vi "Controller Generate Filter Coefficients.vi"(4 "Destination Folder":path, 5 "iwl coeff b":i16=2, 6 "Filter Name":string, 7 "iwl coeff a":i16=2, 8 "Generate FPGA Code?":bool, 9 "wl":i16=20, 10 "denominator":dbl[](array[numeric]), 11 "numerator":dbl[](array[numeric])) -> (1 "gain":dbl, 2 "coeff a":dbl[](array[numeric]), 3 "coeff b":dbl[](array[numeric]))   [LabVIEW 2011]
uses:
  <vilib>/addons/Digital Filter Design/_Objects.llb/DFD Output Iwl Obj.ctl
  <vilib>/addons/Digital Filter Design/_Objects.llb/DFD Quantization Settings.ctl
  <vilib>/addons/Digital Filter Design/_Objects.llb/DFD Quantization Sources.ctl
  <vilib>/addons/Digital Filter Design/_Objects.llb/DFD Phase Setting.ctl
  <vilib>/addons/Digital Filter Design/_Objects.llb/DFD Coef Norm Type.ctl
  <vilib>/addons/Digital Filter Design/FXPModel.llb/DFD FXP Quantize Coef (Advanced).vi
  <vilib>/addons/Digital Filter Design/NI_DigFilterLicensed.lvlib
  <vilib>/addons/Digital Filter Design/CodeGen.llb/DFD FXP LabVIEW FPGA Code Generator.vi
panel:
  out "max gain error (dB)":dbl
  out "max phase error (deg)":dbl
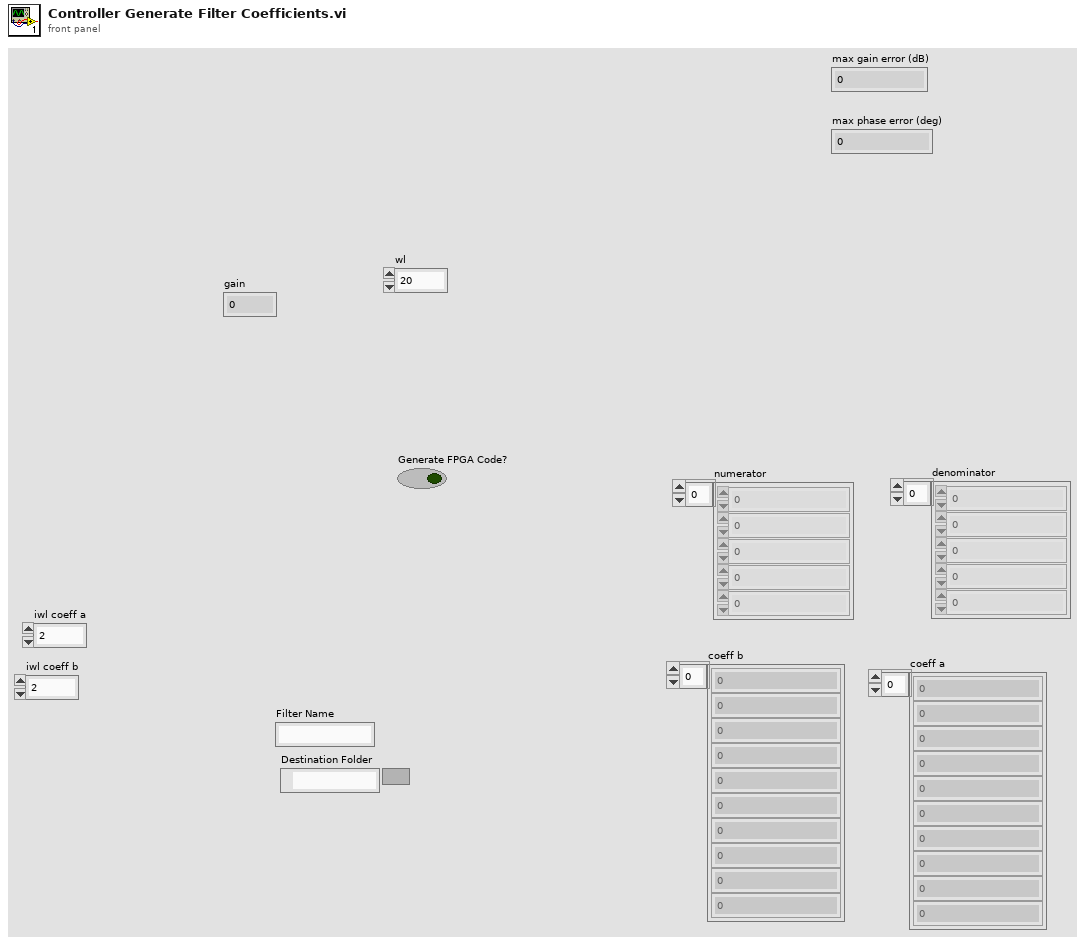
[diagram p1: front panel]
types:
  T1 = typedef "NI_DigFilterLicensed.lvlib/DFD Coef Norm Type.ctl" = enum16{"No Norm", "Time Domain 1-Norm", "Time Domain 2-Norm", "Time Domain Inf-Norm"}
  T2 = typedef "NI_DigFilterLicensed.lvlib/DFD Phase Setting.ctl" = cluster{"unwrap? (F)":bool, "degree? (F)":bool}
  T3 = typedef "NI_DigFilterLicensed.lvlib/DFD Quantization Settings.ctl" = cluster{"source":T4, "wl":i16, "iwl":i16, "overflow mode":enum16{"Saturation", "Wrap"}, "rounding mode":enum16{"Nearest", "Truncation"}, "signed?":bool}
  T4 = typedef "NI_DigFilterLicensed.lvlib/DFD Quantization Sources.ctl" = u16
  T5 = typedef "NI_DigFilterLicensed.lvlib/DFD Output Iwl Obj.ctl" = cluster{"output option":enum16{"Auto", "Same As Input", "User Defined"}, "integer word length":i16}
  T6 = typedef "NI_DigFilterLicensed.lvlib/DFD Filter Obj.ctl" = cluster{"mSRate_Fs":dbl, "mSRate_Version":string, "mSRate_Comments":string, "mSRate_OrgCoef":T7, "mSRate_CurCoef":T7, "mSRate_Quantized?":bool, "mSRate_QCoef":T7, "mSRate_QSettings":T9[], "mSRate_Order":i32, "mSRate_Scaling":cluster{"mSRate_ScaleByPowerOf2?":bool, "mSRate_ScaleType":T1}}
  T7 = typedef "NI_DigFilterLicensed.lvlib/DFD Filter Coef.ctl" = cluster{"type":T8, "gain":dbl, "coef a (k)":dbl[], "coef b (v)":dbl[]}
  T8 = typedef "NI_DigFilterLicensed.lvlib/DFD Filter Structure Type Selector.ctl" = enum16{"Undefined", "FIR Direct Form", "FIR Direct Form Transposed", "FIR Symmetric", "FIR Antisymmetric", "IIR Direct Form I", "IIR Direct Form I Transposed", "IIR Direct Form II", "IIR Direct Form II Transposed", "IIR Cascaded Second Order Sections Form I", "IIR Cascaded Second Order Sections Form I Transposed", "IIR Cascaded Second Order Sections Form II", "IIR Cascaded Second Order Sections Form II Transposed", "Lattice Allpass (basic sections)", "Lattice Allpass (one multiplier sections)", "Lattice Allpass (normalized sections)", "Lattice AR (basic sections)", "Lattice AR (one multiplier sections)", "Lattice AR (normalized sections)", "Lattice MA (minimum phase)", "Lattice MA (maximum phase)", "Lattice ARMA (basic sections)", "Lattice ARMA (one multiplier sections)", "Lattice ARMA (normalized sections)"}
  T9 = typedef "NI_DigFilterLicensed.lvlib/dfd_Internal Quantization Settings.ctl" = cluster{"source":T10, "wl":i16, "iwl":i16, "overflow mode":enum16{"Saturation", "Wrap"}, "rounding mode":enum16{"Nearest", "Truncation"}, "signed?":bool}
  T10 = typedef "NI_DigFilterLicensed.lvlib/dfd_Internal Quantization Srcs.ctl" = u16
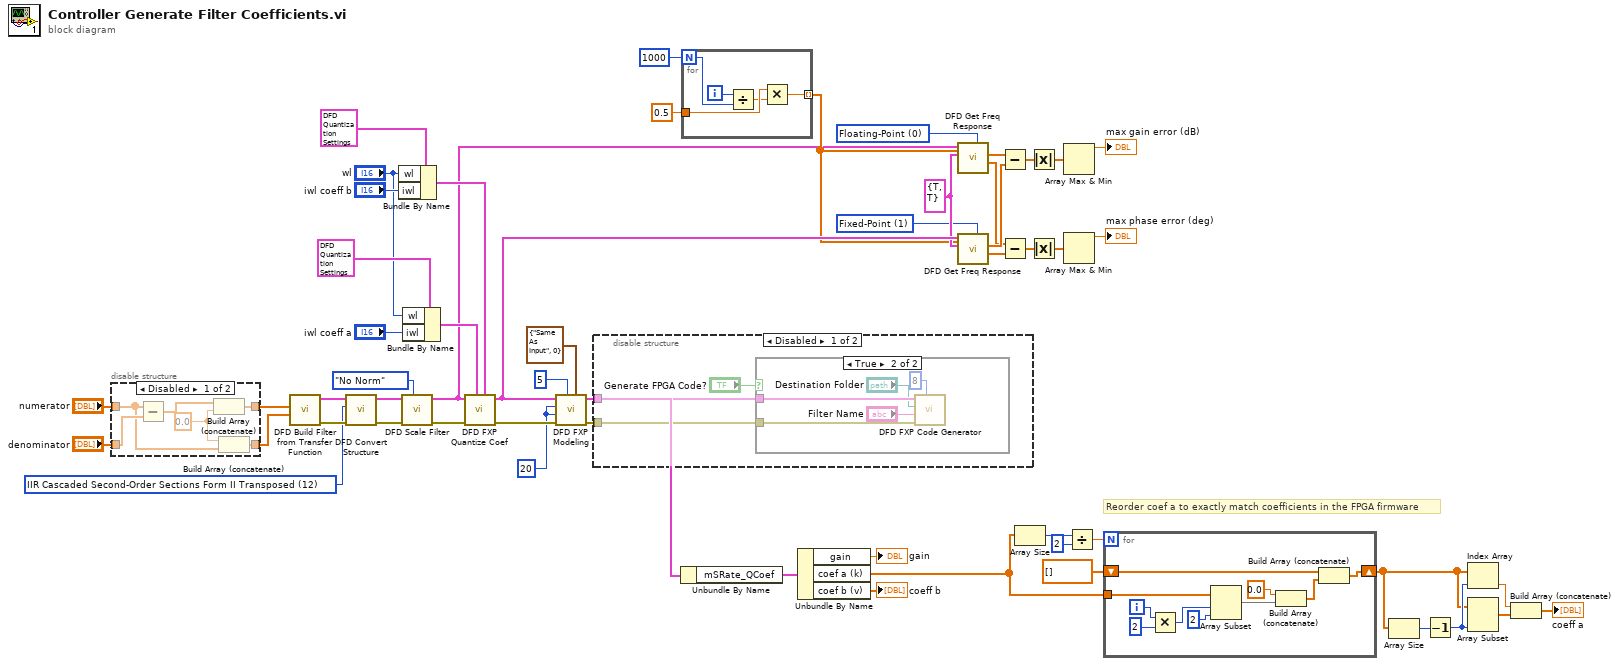
[diagram p0: block diagram]
diagram:
  w34 = u16 0 items=["Floating-Point", "Fixed-Point"] ("output option")
  w42 = u16 1 items=["Floating-Point", "Fixed-Point"] ("output option")
  w43 = T2 {"unwrap? (F)"=TRUE, "degree? (F)"=TRUE} ("phase view")
  w47 = i16 20 ("input word length")
  w54 = u16 12 items=["FIR Direct Form"=1, "FIR Direct Form Transposed"=2, "FIR Symmetric"=3, "FIR Antisymmetric"=4, "IIR Direct Form I"=5, "IIR Direct Form I Transposed"=6, "IIR Direct Form II"=7, "IIR Direct Form II Transposed"=8, "IIR Cascaded Second-Order Sections Form I"=9, "IIR Cascaded Second-Order Sections Form I Transposed"=10, "IIR Cascaded Second-Order Sections Form II"=11, "IIR Cascaded Second-Order Sections Form II Transposed"=12, "Lattice Allpass (basic sections)"=13, "Lattice Allpass (one multiplier sections)"=14, "Lattice Allpass (normalized sections)"=15, "Lattice AR (basic sections)"=16, "Lattice AR (one multiplier sections)"=17, "Lattice AR (normalized sections)"=18, "Lattice MA (minimum phase)"=19, "Lattice MA (maximum phase)"=20, "Lattice ARMA (basic sections)"=21, "Lattice ARMA (one multiplier sections)"=22, "Lattice ARMA (normalized sections)"=23] ("target structure")
  # "Reorder coef a to exactly match coefficients in the FPGA firmware"
  n1 = disable-structure shown="Disabled" {
    disable-tunnel: "denominator" -> [w62 w63]
    disable-tunnel: "numerator" -> [w60 w64]
    disable-tunnel: [w58 w64] -> w3
    disable-tunnel: [w57 w63] -> w2
    frame Disabled {
      w59 = 0.0 ("Numeric")
      n2 = Subtract(x=w60, y=w62) -> (x-y=w61:dbl[])
      n3 = Build Array (concatenate)(w61, w59) -> (w58:dbl[])
      n4 = Build Array (concatenate)(w59, w60) -> (w57:dbl[])
    }
    frame Enabled {
    }
  }
  n5 = call <vilib>:"DFD Build Filter from Transfer Function.vi"("denominator"=w2, "numerator"=w3) -> ("error out"=w55:errorcluster, "filter out"=w49:T6)  [unwired: 8 in]
  n6 = call <vilib>:"DFD Convert Structure.vi"("error in (no error)"=w55, "target structure"=w54, "filter in"=w49) -> ("error out"=w18:errorcluster, "filter out"=w19:T6)  [unwired: 7 in]
  n7 = Bundle By Name(cluster=T3 {"source"=7, "wl"=20, "iwl"=1, "overflow mode"=enum."Saturation", "rounding mode"=enum."Nearest", "signed?"=TRUE} ("coefficients b/v quantizer"), "wl"="wl", "iwl"="iwl coeff b") -> (w36:T3)
  n8 = call <vilib>:"DFD Scale Filter.vi"("scale type"=DFD_Coef_Norm_Type."No Norm", "error in (no error)"=w18, "filter in"=w19) -> ("error out"=w17:errorcluster, "filter out"=w16:T6)  [unwired: 7 in]
  n9 = Bundle By Name(cluster=T3 {"source"=0, "wl"=20, "iwl"=1, "overflow mode"=enum."Saturation", "rounding mode"=enum."Nearest", "signed?"=TRUE} ("coefficients a/k quantizer"), "wl"="wl", "iwl"="iwl coeff a") -> (w35:T3)
  n10 = call-poly <vilib>:"DFD FXP Quantize Coef.vi"("coefficients b/v quantizer"=w36, "coefficients a/k quantizer"=w35, "error in (no error)"=w17, "filter in"=w16) -> ("error out"=w53:errorcluster, "filter out"=w44:T6)  [unwired: 6 in]
  n11 = call <vilib>:"DFD FXP Modeling.vi"("output integer word length"=T5 {"output option"=enum."Same As Input", "integer word length"=0}, "input integer word length"=i16 5, "error in (no error)"=w53, "output word length"=w47, "input word length"=w47, "filter in"=w44) -> ("error out"=w56:errorcluster, "filter out"=w45:T6)  [unwired: 4 in]
  n12 = disable-structure shown="Disabled" {
    disable-tunnel: w56 -> [w67 _]
    disable-tunnel: w45 -> [w66 _]
    frame Disabled {
      n13 = case shown="True" "Generate FPGA Code?" {
        tunnel: w67 -> [_ w72]
        tunnel: w66 -> [_ w71]
        frame False {
        }
        frame True {
          n14 = call-poly <vilib>:"DFD FXP Code Generator.vi"("# channels"=8, "error in (no error)"=w72, "filter name"="Filter Name", "destination folder"="Destination Folder", "filter in"=w71) -> ()  [unwired: 2 in, 5 out]
        }
      }
    }
    frame Enabled {
    }
  }
  n15 = Unbundle By Name(w45) -> ("mSRate_QCoef"=w52:T7)
  n16 = for {
    N: 1000 -> [w76]
    tunnel: 0.5 -> [w75]
    tunnel: [w73] -> w29 mode=indexing
    i -> [w77]
    n17 = Divide(x=w77, y=w76) -> (x/y=w74:dbl)
    n18 = Multiply(x=w75, y=w74) -> (x*y=w73:dbl)
  }
  n19 = Unbundle By Name(w52) -> ("gain"=→"gain":dbl, "coef a (k)"=w11:dbl[], "coef b (v)"=→"coeff b":dbl[])
  n20 = call <vilib>:"DFD Get Freq Response.vi"("output option"=w34, "freq points [Hz]"=w29, "phase view"=w43, "filter in"=w16) -> ("phase"=w31:dbl[], "magnitude"=w33:dbl[])  [unwired: 4 in, 2 out]
  n21 = call <vilib>:"DFD Get Freq Response.vi"("output option"=w42, "freq points [Hz]"=w29, "phase view"=w43, "filter in"=w44) -> ("phase"=w30:dbl[], "magnitude"=w32:dbl[])  [unwired: 4 in, 2 out]
  n22 = Subtract(x=w33, y=w32) -> (x-y=w27:dbl[])
  n23 = Subtract(x=w31, y=w30) -> (x-y=w24:dbl[])
  n24 = Array Size(array=w11) -> (size(s)=w10:i32)
  n25 = Absolute Value(x=w27) -> (abs(x)=w26:dbl[])
  n26 = Absolute Value(x=w24) -> (abs(x)=w25:dbl[])
  n27 = Array Max & Min(array=w26) -> (max value=→"max gain error (dB)":dbl)  [unwired: 3 out]
  n28 = Array Max & Min(array=w25) -> (max value=→"max phase error (deg)":dbl)  [unwired: 3 out]
  n29 = Divide(x=w10, y=2) -> (x/y=w13:dbl)
  n30 = for {
    N: w13 -> [_]
    tunnel: w11 -> [w80]
    shift-right: [w78] -> w5
    shift-left: dbl[] [] ("coef a (k)") -> [w79]
    i -> [w87]
    n31 = Multiply(x=w87, y=2) -> (x*y=w85:i32)
    n32 = Array Subset(array=w80, index=w85, length=2) -> (w83:dbl[])
    n33 = Build Array (concatenate)(0.0 ("x/y"), w83) -> (w81:dbl[])
    n34 = Build Array (concatenate)(w79, w81) -> (w78:dbl[])
  }
  n35 = Array Size(array=w5) -> (size(s)=w4:i32)
  n36 = Decrement(x=w4) -> (x-1=w8:i32)
  n37 = Index Array(array=w5, index=w8) -> (element=w7:dbl)
  n38 = Array Subset(array=w5, length=w8) -> (w6:dbl[])  [unwired: 1 in]
  n39 = Build Array (concatenate)(w7, w6) -> (→"coeff a":dbl[])
